vi "arrayMath.vi"() -> ()   [LabVIEW 2020]
panel:
  out "x+y":dbl[](array[numeric])
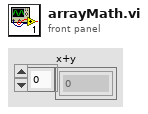
[diagram p1: front panel]
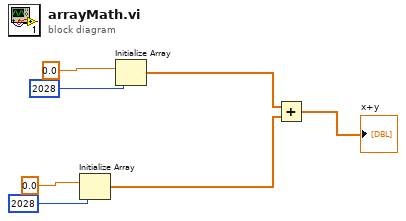
[diagram p0: block diagram]
diagram:
  n1 = Initialize Array(0.0 ("element"), 2028 ("dimension size")) -> (w3:dbl[])
  n2 = Initialize Array(0.0 ("element"), 2028 ("dimension size")) -> (w2:dbl[])
  n3 = Add(x=w2, y=w3) -> (x+y=→"x+y":dbl[])
